vi "niDAQmx Write (Digital Bool 1Line 1Point).vi"(0 "task in":refnum<class "Session Factory.lvclass">, 1 "auto start":bool=TRUE, 7 "data":bool, 9 "timeout":dbl=10.0 format="%0.2f", 11 "error in":errorcluster) -> (4 "task out":refnum<class "Session Factory.lvclass">, 10 "number of samples written per channel":u32, 15 "error out":errorcluster)   [LabVIEW 2021, in "Session Management niDAQmx.lvlib" / "Session Factory.lvclass"]
doc: "Writes a single Boolean sample to a task that contains a digital output channel composed of a single line."
uses:
  Session Factory.lvclass
  NI_DAQmx_client/RPC Messages/nidaqmx_grpc_WriteDigitalLinesRequest.ctl
  NI_DAQmx_client/RPC Messages/nidevice_grpc_Session.ctl
  NI_DAQmx_client/RPC Messages/nidevice_grpc_Session_session/nidevice_grpc_Session_session.lvclass
  NI_DAQmx_client/RPC Messages/nidaqmx_grpc_WriteDigitalLinesRequest_data_layout_enum/nidaqmx_grpc_WriteDigitalLinesRequest_data_layout_enum.lvclass
  NI_DAQmx_client/RPC Messages/nidaqmx_grpc_GroupBy.ctl
  NI_DAQmx_client/RPC Messages/nidaqmx_grpc_WriteDigitalLinesRequest_data_layout_enum/nidaqmx_grpc_WriteDigitalLinesRequest_data_layout_enum.lvclass/nidaqmx_grpc_WriteDigitalLinesRequest_data_layout_enum.ctl
  Session Factory.lvclass/Session Factory.ctl
  NI_DAQmx_client/NI_DAQmx_client.lvlib
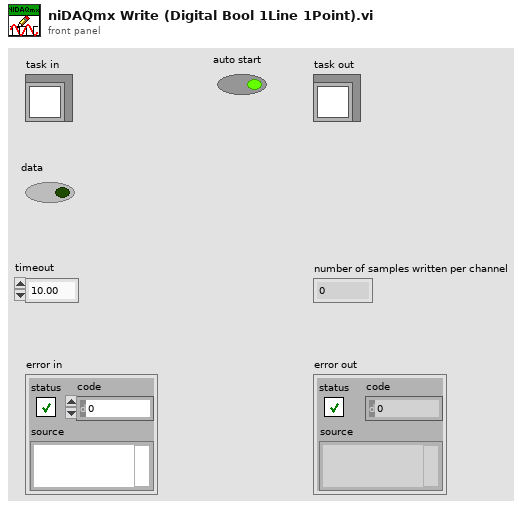
[diagram p1: front panel]
types:
  T1 = typedef "NI_DAQmx_client.lvlib/nidaqmx_grpc_GroupBy.ctl" = enum32{"GROUP_BY_GROUP_BY_CHANNEL", "GROUP_BY_GROUP_BY_SCAN_NUMBER"}
  T2 = typedef "NI_DAQmx_client.lvlib/nidaqmx_grpc_WriteDigitalLinesRequest.ctl" = cluster{"task":T3, "num_samps_per_chan":i32, "auto_start":bool, "timeout":dbl, "nidaqmx_grpc_WriteDigitalLinesRequest_data_layout_enum":refnum<class "nidaqmx_grpc_WriteDigitalLinesRequest_data_layout_enum.lvclass">, "write_array":u8[]}
  T3 = typedef "NI_DAQmx_client.lvlib/nidevice_grpc_Session.ctl" = cluster{"nidevice_grpc_Session_session":refnum<class "nidevice_grpc_Session_session.lvclass">}
  T4 = typedef "grpc-lvsupport-release.lvlib/grpcId.ctl" = u64
  T5 = typedef "NI_DAQmx_client.lvlib/nidaqmx_grpc_WriteDigitalLinesResponse.ctl" = cluster{"status":i32, "samps_per_chan_written":i32}
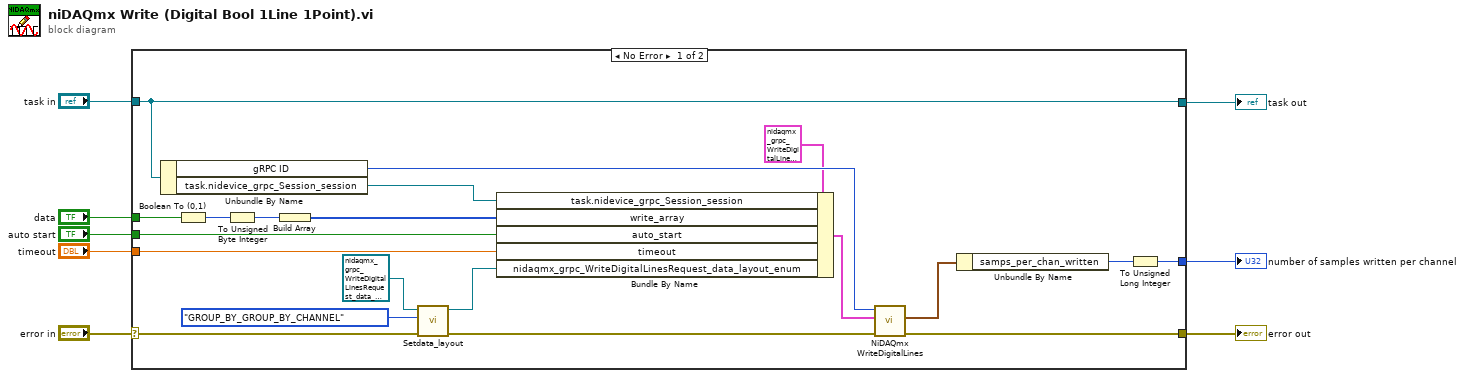
[diagram p0: block diagram]
diagram:
  n1 = case shown="No Error" "error in" {
    selector: "error in" -> [w13 w30]
    tunnel: [w28 w30] -> w7
    tunnel: "task in" -> [w27 w29]
    tunnel: [w27 w29] -> w5
    tunnel: "auto start" -> [w23 _]
    tunnel: "data" -> [w20 _]
    tunnel: "timeout" -> [w21 _]
    tunnel: [w14 _] -> w1
    frame No Error {
      n2 = Unbundle By Name(w27) -> ("gRPC ID"=w26:T4, "task.nidevice_grpc_Session_session"=w24:refnum<class "nidevice_grpc_Session_session.lvclass">)
      n3 = Boolean To (0,1)(Boolean=w20) -> (0, 1=w19:i16)
      n4 = To Unsigned Byte Integer(number=w19) -> (unsigned 8bit integer=w18:u8)
      n5 = Build Array(w18) -> (w17:u8[])
      n6 = call "Setdata_layout.vi"("error in (no error)"=w13, "Set_Val"=nidaqmx_grpc_GroupBy."GROUP_BY_GROUP_BY_CHANNEL", "OneOfTemplate in"=refnum<class "nidaqmx_grpc_WriteDigitalLinesRequest_data_layout_enum.lvclass"> refnum ("nidaqmx_grpc_WriteDigitalLinesRequest_data_layout_enum")) -> ("error out"=w12:errorcluster, "OneOfTemplate out"=w9:refnum<class "nidaqmx_grpc_WriteDigitalLinesRequest_data_layout_enum.lvclass">)  [unwired: 7 in]
      n7 = Bundle By Name(cluster=T2 {"task"={"nidevice_grpc_Session_session"=refnum}, "num_samps_per_chan"=0, "auto_start"=FALSE, "timeout"=0.0, "nidaqmx_grpc_WriteDigitalLinesRequest_data_layout_enum"=refnum, "write_array"=[]} ("Request Data"), "task.nidevice_grpc_Session_session"=w24, "write_array"=w17, "auto_start"=w23, "timeout"=w21, "nidaqmx_grpc_WriteDigitalLinesRequest_data_layout_enum"=w9) -> (w22:T2)
      n8 = call "NiDAQmx WriteDigitalLines.vi"("error in"=w12, "Request Data"=w22, "gRPC ID"=w26) -> ("error out"=w28:errorcluster, "Response Data"=w16:T5)  [unwired: 6 in, 1 out]
      n9 = Unbundle By Name(w16) -> ("samps_per_chan_written"=w15:i32)
      n10 = To Unsigned Long Integer(number=w15) -> (unsigned 32bit integer=w14:u32)
    }
    frame Error {
    }
  }
  "error out" <- w7
  "task out" <- w5
  "number of samples written per channel" <- w1
